vi "Simulator Release.vi"(7 "Module Name":string, 8 "error in (no error)":errorcluster) -> (0 "error out":errorcluster)   [LabVIEW 2019, in "ADLINK Motion Card.lvlib"]
uses:
  ADLINK Motion Card.lvlib
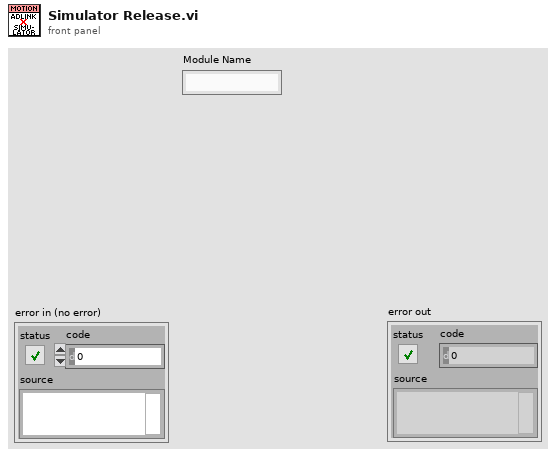
[diagram p1: front panel]
types:
  T1 = typedef "ADLINK Motion Card.lvlib/SEQ Data.ctl" = cluster{"Current Position":dbl, "Target Position":dbl, "Velocity":dbl, "Acceleration":dbl, "Arrived?":bool, "data value reference":refnum<data-value>, "VI Refnum":refnum<vi>}
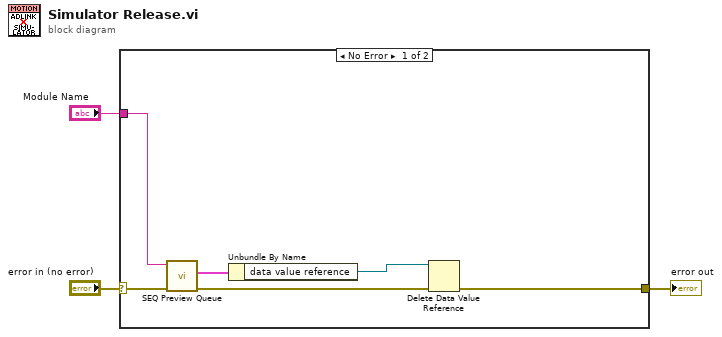
[diagram p0: block diagram]
diagram:
  n1 = case shown="No Error" "error in (no error)" {
    selector: "error in (no error)" -> [w8 w10]
    tunnel: [w4 w10] -> w3
    tunnel: "Module Name" -> [w9 _]
    frame No Error {
      n2 = call "SEQ Preview Queue.vi"("error in (no error)"=w8, "Queue Name"=w9) -> ("error out"=w6:errorcluster, "Setting"=w7:T1)  [unwired: 8 in]
      n3 = Unbundle By Name(w7) -> ("data value reference"=w5:refnum<data-value>)
      n4 = Delete Data Value Reference(data value reference=w5, error in=w6) -> (error out=w4:errorcluster)  [unwired: 1 out]
    }
    frame Error {
    }
  }
  "error out" <- w3
